vi "Scope_packet_encoder.vi"(11 "Scope settings":T1={"run_stop"=FALSE, "single mode"=FALSE, "Trigger mode"=enum."Rising Edge", "Trigger source"=0, "trigger level"=0.0, "acq width"=100.0} {"Trigger source" items=["VLa", "VLb", "VLc"]; "acq width" min=-12.0 max=12.0 step=1.0; "trigger level" min=-12.0 max=12.0 step=1.0}) -> (3 "concatenated string":string)   [LabVIEW 2015, in "Hardware.lvlib"]
uses:
  Hardware.lvlib
  Settings/Scope settings.ctl
  Settings/Settings.lvlib
panel:
  out "unsigned 32bit integer":u32 format="%x"
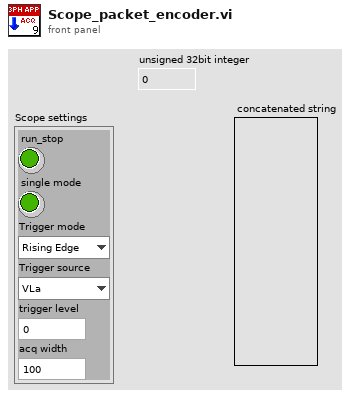
[diagram p1: front panel]
types:
  T1 = typedef "Settings.lvlib/Scope settings.ctl" = cluster{"run_stop":bool, "single mode":bool, "Trigger mode":enum16{"Auto", "Rising Edge", "Falling Edge", "Both Edges"}, "Trigger source":u16, "trigger level":dbl, "acq width":dbl}
  T2 = enum16{"big-endian, network order", "native, host order", "little-endian"}
  T3 = enum16{"Auto", "Rising Edge", "Falling Edge", "Both Edges"}
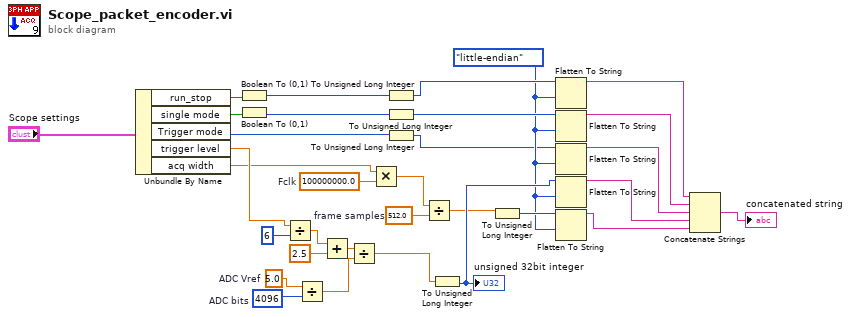
[diagram p0: block diagram]
diagram:
  w1 = 512.0  # frame samples
  w17 = 100000000.0  # Fclk
  w24 = 5.0  # ADC Vref
  w23 = u32 4096  # ADC bits
  w6 = T2."little-endian" ("byte order (0:big-endian, network order)")
  n1 = Unbundle By Name("Scope settings") -> ("run_stop"=w15:bool, "single mode"=w14:bool, "Trigger mode"=w10:T3, "trigger level"=w20:dbl, "acq width"=w16:dbl)
  n2 = Boolean To (0,1)(Boolean=w15) -> (0, 1=w11:i16)
  n3 = Boolean To (0,1)(Boolean=w14) -> (0, 1=w9:i16)
  n4 = Divide(x=w20, y=u32 6) -> (x/y=w26:dbl)
  n5 = Divide(x=w24, y=w23) -> (x/y=w21:dbl)
  n6 = Add(x=w26, y=2.5) -> (x+y=w22:dbl)
  n7 = Divide(x=w22, y=w21) -> (x/y=w4:dbl)
  n8 = Multiply(x=w16, y=w17) -> (x*y=w2:dbl)
  n9 = To Unsigned Long Integer(number=w11) -> (unsigned 32bit integer=w8:u32)
  n10 = To Unsigned Long Integer(number=w9) -> (unsigned 32bit integer=w7:u32)
  n11 = To Unsigned Long Integer(number=w10) -> (unsigned 32bit integer=w5:u32)
  n12 = Divide(x=w2, y=w1) -> (x/y=w3:dbl)
  n13 = To Unsigned Long Integer(number=w4) -> (unsigned 32bit integer=w19:u32)
  "unsigned 32bit integer" <- w19
  n14 = To Unsigned Long Integer(number=w3) -> (unsigned 32bit integer=w18:u32)
  n15 = Flatten To String(anything=w8, byte order (0:big-endian, network order)=w6) -> (data string=w13:string)  [unwired: 2 in, 2 out]
  n16 = Flatten To String(anything=w7, byte order (0:big-endian, network order)=w6) -> (data string=w12:string)  [unwired: 2 in, 2 out]
  n17 = Flatten To String(anything=w5, byte order (0:big-endian, network order)=w6) -> (data string=w32:string)  [unwired: 2 in, 2 out]
  n18 = Flatten To String(anything=w19, byte order (0:big-endian, network order)=w6) -> (data string=w30:string)  [unwired: 2 in, 2 out]
  n19 = Flatten To String(anything=w18, byte order (0:big-endian, network order)=w6) -> (data string=w29:string)  [unwired: 2 in, 2 out]
  n20 = Concatenate Strings(w13, w12, w32, w30, w29) -> (→"concatenated string":string)
